vi "getSerializedData.vi"(0 "reference":refnum<class "AbstractEdge.lvclass">, 5 "error in (no error)":errorcluster) -> (14 "reference out":refnum<class "AbstractEdge.lvclass">, 15 "startNode":refnum<class "AbstractNode.lvclass">, 16 "endNode":refnum<class "AbstractNode.lvclass">, 17 "xmlOut":string, 19 "error out":errorcluster)   [LabVIEW 2014, in "AbstractEdge.lvclass"]
doc: "Gets data to store"
uses:
  <resource>/Framework/Providers/Open_GDS/UML/AbstractEdge_class/AbstractEdge.lvclass
  <resource>/Framework/Providers/Open_GDS/UML/AbstractNode_class/AbstractNode.lvclass
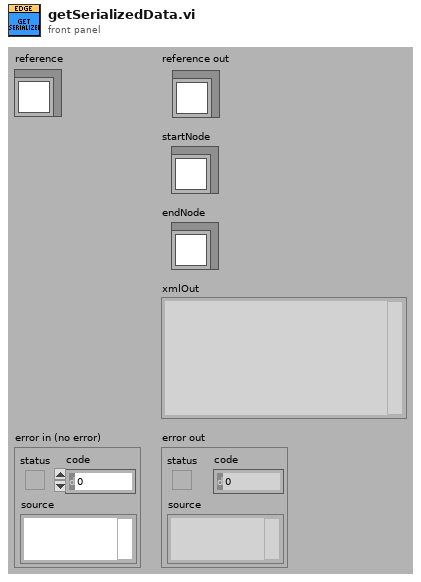
[diagram p1: front panel]
types:
  T1 = typedef "AbstractEdge.lvclass/ObjectAttributes.ctl" = cluster{"start":refnum<class "AbstractNode.lvclass">, "end":refnum<class "AbstractNode.lvclass">}
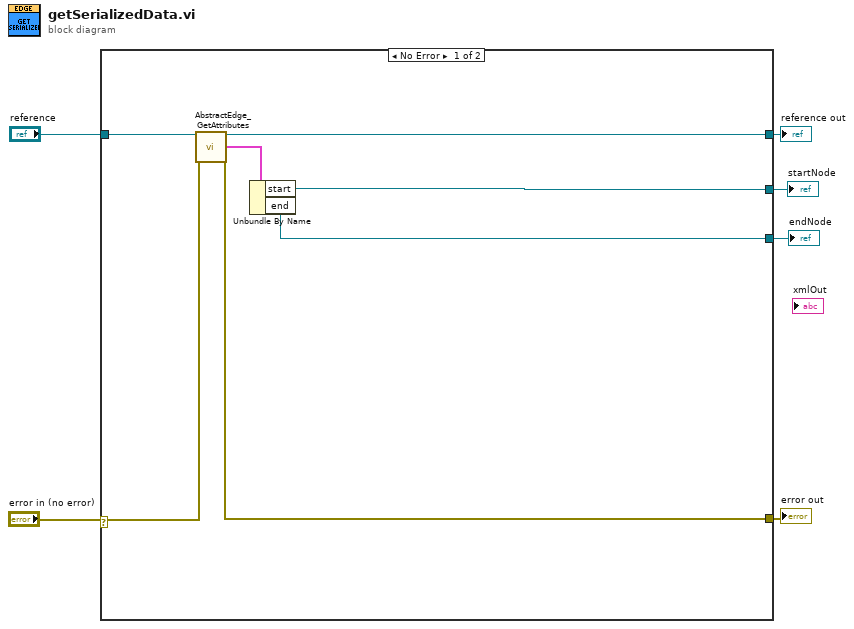
[diagram p0: block diagram]
diagram:
  n1 = case shown="No Error" "error in (no error)" {
    selector: "error in (no error)" -> [w10 w14]
    tunnel: "reference" -> [w13 w15]
    tunnel: [w12 w14] -> w5
    tunnel: [w11 w15] -> w4
    tunnel: [w9 _] -> w2
    tunnel: [w8 _] -> w1
    frame No Error {
      n2 = call <resource>:"AbstractEdge_GetAttributes.vi"("reference in"=w13, "error in (no error)"=w10) -> ("reference out"=w11:refnum<class "AbstractEdge.lvclass">, "Data"=w7:T1, "error out"=w12:errorcluster)  [unwired: 1 in, 14 out]
      n3 = Unbundle By Name(w7) -> ("start"=w9:refnum<class "AbstractNode.lvclass">, "end"=w8:refnum<class "AbstractNode.lvclass">)
    }
    frame Error {
    }
  }
  "reference out" <- w4
  "error out" <- w5
  "startNode" <- w2
  "endNode" <- w1
